vi "FedorPowerUp.vi"(8 "error in (no error)":errorcluster, 10 "DAQmx Device Name":tag="6251") -> (0 "error out":errorcluster)   [LabVIEW 2015]
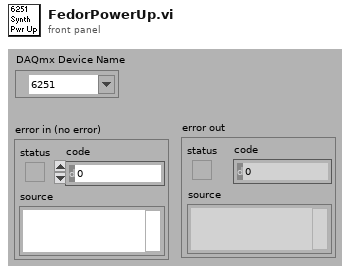
[diagram p1: front panel]
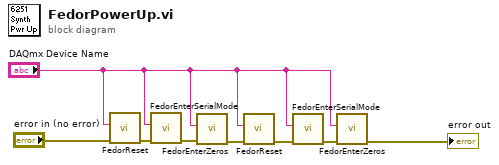
[diagram p0: block diagram]
diagram:
  n1 = call "FedorReset.vi"("error in (no error)"="error in (no error)", "DAQmx Device Name"="DAQmx Device Name") -> ("error out"=w5:errorcluster)  [unwired: 9 out]
  n2 = call "FedorEnterSerialMode.vi"("error in (no error)"=w5, "DAQmx Device Name"="DAQmx Device Name") -> ("error out"=w7:errorcluster)  [unwired: 9 out]
  n3 = call "FedorEnterZeros.vi"("error in (no error)"=w7, "DAQmx Device Name"="DAQmx Device Name") -> ("error out"=w6:errorcluster)  [unwired: 9 out]
  n4 = call "FedorReset.vi"("error in (no error)"=w6, "DAQmx Device Name"="DAQmx Device Name") -> ("error out"=w4:errorcluster)  [unwired: 9 out]
  n5 = call "FedorEnterSerialMode.vi"("error in (no error)"=w4, "DAQmx Device Name"="DAQmx Device Name") -> ("error out"=w3:errorcluster)  [unwired: 9 out]
  n6 = call "FedorEnterZeros.vi"("error in (no error)"=w3, "DAQmx Device Name"="DAQmx Device Name") -> ("error out"=→"error out":errorcluster)  [unwired: 9 out]
